vi "Begin.vi"(11 "Image Size":T1=enum."160x120") -> (0 "error out":errorcluster)   [LabVIEW 2012]
doc: "Called before other user functions, this VI is expected to open initial I/O refnums, load in file data, and do all program initialization. Notice that the <B>error out</B> terminal is simply used for data flow. Wiring it to other structures or subVIs ensures that this VI runs first."
uses:
  <vilib>/Rock Robotics/WPI/Camera/WPI_CameraImageSize.ctl
  <vilib>/Rock Robotics/SystemInterfaces/DIO/FPGA_DIOPWMChannel.ctl
  <vilib>/Rock Robotics/WPI/Camera/WPI_CameraWhite Balance Values.ctl
  <vilib>/Rock Robotics/WPI/Camera/WPI_CameraExposure Values.ctl
  <vilib>/Rock Robotics/WPI/Camera/WPI_CameraFrameRate.ctl
  <vilib>/Rock Robotics/WPI/SafetyOutput/WPI_SafetyOutputConfigMenu.ctl
  <vilib>/Rock Robotics/WPI/DriverStation/WPI_DriverStationRobotMode2.ctl
  <vilib>/Rock Robotics/WPI/Joystick/WPI_JoystickDeviceEnum.ctl
  <vilib>/Rock Robotics/SystemInterfaces/Typedef/FPGA_TypedefSolenoidModule.ctl
  <vilib>/Rock Robotics/WPI/Solenoid/WPI_SolenoidChannel.ctl
  <vilib>/Rock Robotics/SystemInterfaces/DIO/FPGA_DIOChannel.ctl
  <vilib>/Rock Robotics/WPI/Encoder/WPI_EncoderType.ctl
  <vilib>/Rock Robotics/SystemInterfaces/Typedef/FPGA_TypedefDigitalModule.ctl
  <vilib>/Rock Robotics/SystemInterfaces/DIO/FPGA_DIORelayChannel.ctl
  <vilib>/Rock Robotics/WPI/RobotDrive/WPI_RobotDriveOpen2MotorWithJaguar.vi
  Robot Global Data.vi
  <vilib>/Rock Robotics/WPI/Solenoid/WPI_SolenoidOpenSingle.vi
  <vilib>/Rock Robotics/WPI/Counter/WPI_CounterDigitalInputToDigitalSource.vi
  <vilib>/Rock Robotics/WPI/MotorControl/WPI_MotorControlOpen Talon.vi
  <vilib>/Rock Robotics/WPI/Compressor/WPI_CompressorGetSetRefNum.vi
panel:
  out "1699-preferences.ini":string[][](array[string])
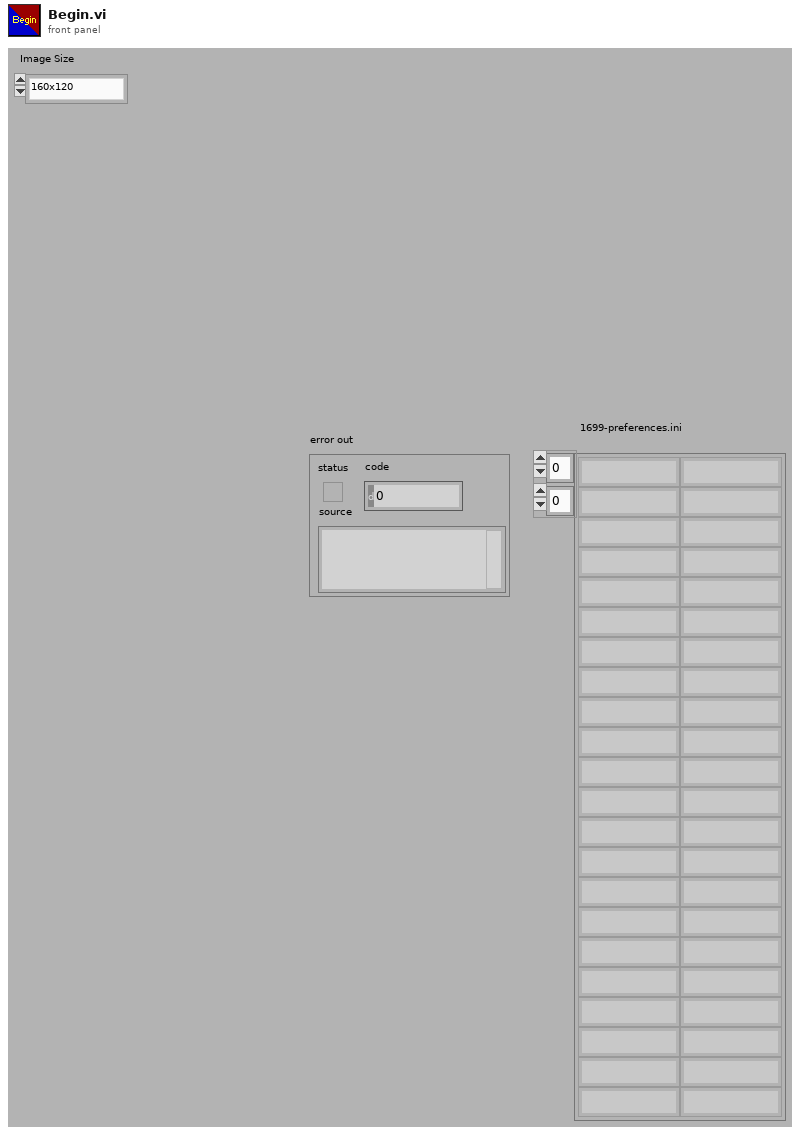
[diagram p1: front panel]
types:
  T1 = typedef "WPI_CameraImageSize.ctl" = enum16{"640x480", "320x240", "160x120"}
  T2 = typedef "FPGA_TypedefDigitalModule.ctl" = enum16{"Digital Module 1", "Digital Module 2"}
  T3 = typedef "FPGA_DIOPWMChannel.ctl" = enum8{"PWM 1", "PWM 2", "PWM 3", "PWM 4", "PWM 5", "PWM 6", "PWM 7", "PWM 8", "PWM 9", "PWM 10", "Invalid"}
  T4 = typedef "FPGA_DIORelayChannel.ctl" = enum8{"Relay 1", "Relay 2", "Relay 3", "Relay 4", "Relay 5", "Relay 6", "Relay 7", "Relay 8", "Invalid"}
  T5 = typedef "FPGA_DIOChannel.ctl" = enum8{"DIO 1", "DIO 2", "DIO 3", "DIO 4", "DIO 5", "DIO 6", "DIO 7", "DIO 8", "DIO 9", "DIO 10", "DIO 11", "DIO 12", "DIO 13", "DIO 14", "Invalid"}
  T6 = typedef "WPI_EncoderType.ctl" = enum16{"1x", "2x", "4x"}
  T7 = typedef "WPI_SolenoidChannel.ctl" = enum8{"Solenoid 1", "Solenoid 2", "Solenoid 3", "Solenoid 4", "Solenoid 5", "Solenoid 6", "Solenoid 7", "Solenoid 8", "Invalid"}
  T8 = typedef "FPGA_TypedefSolenoidModule.ctl" = enum16{"Solenoid Module 1", "Solenoid Module 2"}
  T9 = typedef "WPI_JoystickDeviceEnum.ctl" = enum16{"USB 1", "USB 2", "USB 3", "USB 4", "Kinect 1", "Kinect 2"}
  T10 = typedef "WPI_DriverStationRobotMode2.ctl" = enum16{"Autonomous Disabled", "Autonomous Enabled", "Teleop Disabled", "Teleop Enabled", "Timeout", "Finish", "Test Disabled", "Test Enabled"}
  T11 = typedef "WPI_SafetyOutputConfigMenu.ctl" = enum16{"Enable", "Disable"}
  T12 = typedef "WPI_CameraFrameRate.ctl" = u32
  T13 = typedef "WPI_CameraExposure Values.ctl" = enum16{"Auto", "Flicker-free 50 Hz", "Flicker-free 60 Hz", "Hold current"}
  T14 = typedef "WPI_CameraWhite Balance Values.ctl" = enum16{"Auto", "Fixed indoor", "Fixed outdoor 1", "Fixed outdoor 2", "Fixed fluorescent 1", "Fixed fluorescent 2", "Hold current"}
  T15 = cluster{"[0]":dbl, "[1]":dbl, "[2]":dbl, "[3]":dbl, "[4]":dbl, "[5]":dbl, "[6]":dbl, "[7]":dbl, "[8]":dbl, "[9]":dbl, "[10]":dbl, "[11]":dbl, "[12]":dbl, "[13]":dbl, "[14]":dbl, "[15]":dbl, "[16]":dbl, "[17]":dbl, "[18]":dbl, "[19]":dbl}
  T16 = typedef "WPI_DigitalInputDevRef.ctl" = cluster{"DevStatus":errorcluster, "DIO Channel":T5, "Digital Module":T2}
  T17 = typedef "FPGA_CounterEncoderSourceConvertionLVSourceType.ctl" = cluster{"DevStatus":errorcluster, "AnalogTriggerMode?":bool, "DigitalMode":cluster{"Digital Module":T2, "DIO Channel":T18}, "AnalogTriggerMode":cluster{"AnalogTriggerIndex":T19, "OutputType":T20}}
  T18 = typedef "FPGA_DIODigitalSourceChannel.ctl" = enum8{"DIO 1", "DIO 2", "DIO 3", "DIO 4", "DIO 5", "DIO 6", "DIO 7", "DIO 8", "DIO 9", "DIO 10", "DIO 11", "DIO 12", "DIO 13", "DIO 14", "Disabled"}
  T19 = typedef "FPGA_AnalogTriggerIndex.ctl" = enum8{"Trig 0", "Trig 1", "Trig 2", "Trig 3", "Trig 4", "Trig 5", "Trig 6", "Trig 7", "Invalid"}
  T20 = typedef "FPGA_AnalogTriggerOutType.ctl" = enum16{"InWindow", "TriggerState", "Rising", "Falling"}
  T21 = typedef "WPI_CompressorDevRef.ctl" = cluster{"DevStatus":errorcluster, "DigitalInputDevRef":T16, "RelayDevRef":T22}
  T22 = typedef "WPI_RelayDevRef.ctl" = cluster{"DevStatus":errorcluster, "Relay Channel":T4, "Digital Module":T2, "Relay Direction":T23}
  T23 = typedef "WPI_RelayDirection.ctl" = enum16{"Both directions", "Forward only", "Reverse only"}
  T24 = typedef "WPI_JoystickDevRef.ctl" = cluster{"Device":T9}
  T25 = typedef "WPI_CameraDevRef.ctl" = cluster{"Camera Address":string, "CameraStatus":errorcluster, "Acquire Image Notifier":refnum<notifier>}
  T26 = typedef "WPI_RobotDriveDevRef.ctl" = cluster{"DevStatus":errorcluster, "Motors[]":T27[], "Square Inputs":bool, "Max Output":dbl, "Isochronous":bool}
  T27 = typedef "WPI_MotorControlDeviceRef.ctl" = cluster{"DeviceStatus":errorcluster, "Type":enum16{"PWM", "CAN"}, "PWM":cluster{"Digital Module":T2, "PWM Channel":T3, "DeadBand":T28}, "CAN":cluster{"Device Number":u8, "Control Mode":T29, "Semaphore":T30, "Max Vout":dbl}, "Invert":bool, "TransformRef":T31, "InvTransformRef":T31}
  T28 = typedef "WPI_PWMDeadband.ctl" = cluster{"Name":string, "maxPositivePwm":i32, "minPositivePwm":i32, "centerPwm":i32, "maxNegativePwm":i32, "minNegativePwm":i32, "angularRange":u16}
  T29 = typedef "WPI_CANJaguar_ControlMode.ctl" = enum8{"Percent VBus", "Current", "Speed", "Position", "Voltage"}
  T30 = typedef "Semaphore RefNum" = refnum<k1>
  T31 = typedef "WPI_PWMTransform_ConPane.ctl" = refnum<vi>
  T32 = typedef "WPI_EncoderDevRef.ctl" = cluster{"DevStatus":errorcluster, "EncoderIndex":T33, "CounterIndex":T34, "DistancePerCount":dbl, "Decoding Type":T6}
  T33 = typedef "FPGA_EncoderIdx.ctl" = enum8{"Enc 0", "Enc 1", "Enc 2", "Enc 3", "Invalid"}
  T34 = typedef "FPGA_CounterCtrSystemIndex.ctl" = enum8{"Ctr 0", "Ctr 1", "Ctr 2", "Ctr 3", "Ctr 4", "Ctr 5", "Ctr 6", "Ctr 7", "Invalid"}
  T35 = typedef "WPI_SolenoidDevRef.ctl" = cluster{"DevStatus":errorcluster, "Solenoid Module":T8, "Forward Solenoid Channel":T7, "Reverse Solenoid Channel":T7}
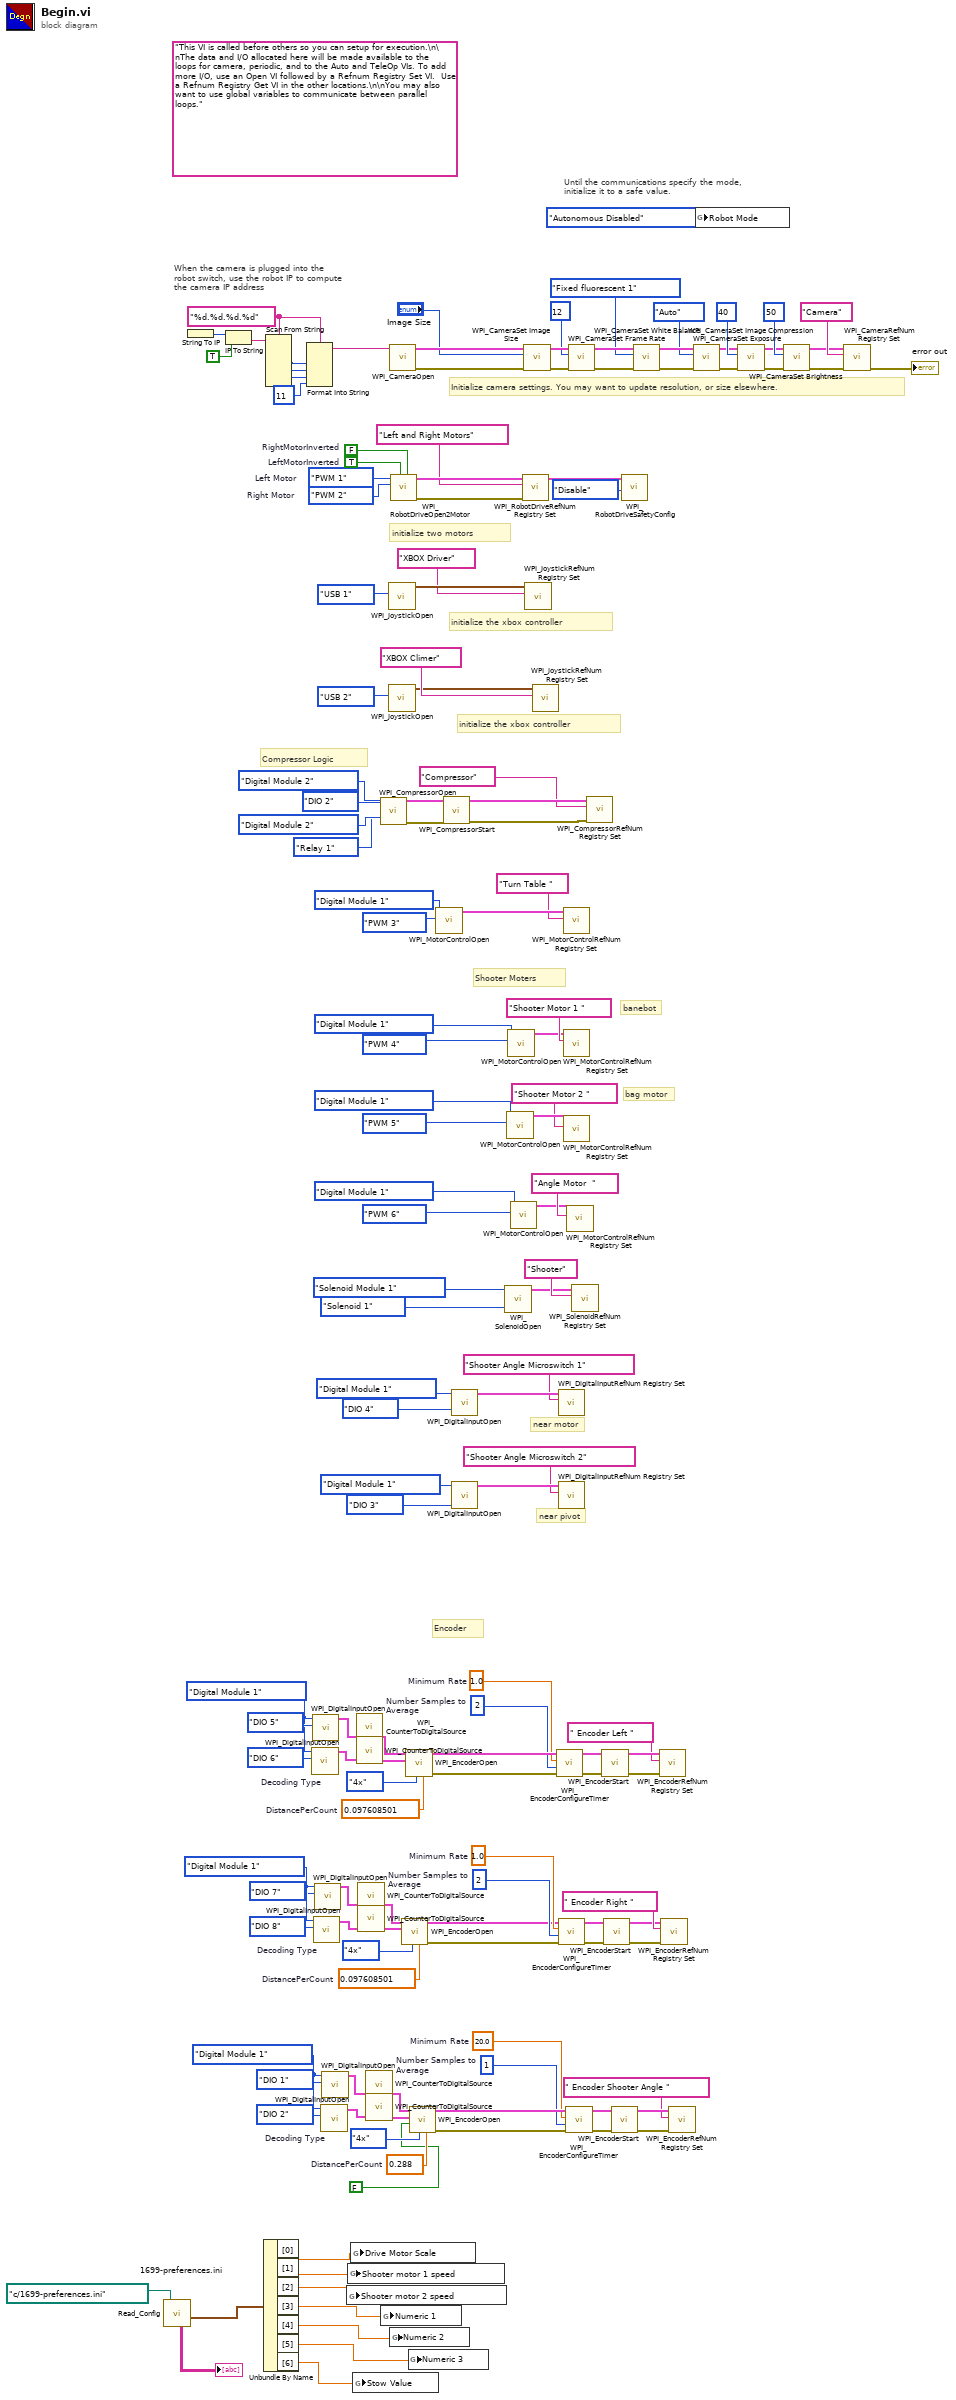
[diagram p0: block diagram]
diagram:
  w45 = FPGA_TypedefDigitalModule."Digital Module 1" ("Digital Module (Module 1)")
  w52 = 0.288  # DistancePerCount
  w53 = WPI_EncoderType."4x"  # Decoding Type
  w54 = u8 1  # Number Samples to Average
  w55 = 20.0  # Minimum Rate
  w80 = FPGA_TypedefDigitalModule."Digital Module 1" ("Digital Module (Module 1)")
  w73 = 0.097608501  # DistancePerCount
  w72 = WPI_EncoderType."4x"  # Decoding Type
  w71 = u8 2  # Number Samples to Average
  w70 = 1.0  # Minimum Rate
  w81 = FPGA_TypedefDigitalModule."Digital Module 1" ("Digital Module (Module 1)")
  w88 = 0.097608501  # DistancePerCount
  w89 = WPI_EncoderType."4x"  # Decoding Type
  w90 = u8 2  # Number Samples to Average
  w91 = 1.0  # Minimum Rate
  w114 = "%d.%d.%d.%d" ("format string")
  (unwired) "This VI is called before others so you can setup for execution.\n\nThe data and I/O allocated here will be made available to the loops for camera, periodic, and to the Auto and TeleOp VIs. To add more I/O, use an Open VI followed by a Refnum Registry Set VI.  Use a Refnum Registry Get VI in the other locations.\n\nYou may also want to use global variables to communicate between parallel loops."
  w125 = FPGA_DIOPWMChannel."PWM 2"  # Right Motor
  w126 = FPGA_DIOPWMChannel."PWM 1"  # Left Motor
  w148 = TRUE  # LeftMotorInverted
  w149 = FALSE  # RightMotorInverted
  # "banebot"
  # "bag motor"
  # "Shooter Moters"
  # "Compressor Logic"
  # "initialize the xbox controller"
  # "near motor"
  # "near pivot"
  # "Encoder"
  # "initialize the xbox controller"
  # "Until the communications specify the mode,\ninitialize it to a safe value."
  # "When the camera is plugged into the\nrobot switch, use the robot IP to compute\nthe camera IP address"
  # "initialize two motors"
  # "Initialize camera settings. You may want to update resolution, or size elsewhere."
  n1 = call "Read_Config.vi"("configuration file path"=path "c:/1699-preferences.ini") -> ("PID Out"=w42:T15, "Array"=→"1699-preferences.ini":string[][])  [unwired: 2 in, 2 out]
  n2 = String To IP() -> (0:w121:u32)  [unwired: 1 in]
  n3 = IP To String(1:TRUE ("dot notation? (F)"), 2:w121) -> (0:w119:string)
  n4 = Unbundle By Name(w42) -> ("[0]"=w41:dbl, "[1]"=w40:dbl, "[2]"=w39:dbl, "[3]"=w38:dbl, "[4]"=w37:dbl, "[5]"=w36:dbl, "[6]"=w35:dbl)
  n5 = Scan From String(format string=w114, input string=w119) -> (output 1=w118:i32, output 2=w117:i32, output 3=w116:i32)  [unwired: 7 in, 3 out]
  n6 = Format Into String(format string=w114, w118, w117, w116, 11 ("Compression")) -> (resulting string=w110:string)  [unwired: 2 in, 1 out]
  n7 = call <vilib>:"WPI_DigitalInputOpen.vi"("DIO Channel"=FPGA_DIOChannel."DIO 6", "Digital Module (Module 1)"=w81) -> ("DigitalInputDevRef"=w85:T16)  [unwired: 8 in, 1 out]
  n8 = call <vilib>:"WPI_DigitalInputOpen.vi"("DIO Channel"=FPGA_DIOChannel."DIO 5", "Digital Module (Module 1)"=w81) -> ("DigitalInputDevRef"=w84:T16)  [unwired: 8 in, 1 out]
  n9 = call <vilib>:"WPI_DigitalInputOpen.vi"("DIO Channel"=FPGA_DIOChannel."DIO 8", "Digital Module (Module 1)"=w80) -> ("DigitalInputDevRef"=w76:T16)  [unwired: 8 in, 1 out]
  n10 = call <vilib>:"WPI_DigitalInputOpen.vi"("DIO Channel"=FPGA_DIOChannel."DIO 7", "Digital Module (Module 1)"=w80) -> ("DigitalInputDevRef"=w77:T16)  [unwired: 8 in, 1 out]
  n11 = call <vilib>:"WPI_DigitalInputOpen.vi"("DIO Channel"=FPGA_DIOChannel."DIO 2", "Digital Module (Module 1)"=w45) -> ("DigitalInputDevRef"=w49:T16)  [unwired: 8 in, 1 out]
  n12 = call <vilib>:"WPI_DigitalInputOpen.vi"("DIO Channel"=FPGA_DIOChannel."DIO 1", "Digital Module (Module 1)"=w45) -> ("DigitalInputDevRef"=w48:T16)  [unwired: 8 in, 1 out]
  n13 = global write "Robot Global Data.vi" "Shooter motor 2 speed"(w39) -> ()
  n14 = global write "Robot Global Data.vi" "Shooter motor 1 speed"(w40) -> ()
  n15 = global write "Robot Global Data.vi" "Drive Motor Scale"(w41) -> ()
  n16 = global write "Robot Global Data.vi" "Stow Value"(w35) -> ()
  n17 = call-poly <vilib>:"WPI_CounterToDigitalSource.vi"("DigitalInputDevRef"=w84) -> ("Digital Source"=w86:T17)  [unwired: 6 in]
  n18 = call-poly <vilib>:"WPI_CounterToDigitalSource.vi"("DigitalInputDevRef"=w85) -> ("Digital Source"=w87:T17)  [unwired: 6 in]
  n19 = call-poly <vilib>:"WPI_CounterToDigitalSource.vi"("DigitalInputDevRef"=w77) -> ("Digital Source"=w75:T17)  [unwired: 6 in]
  n20 = call-poly <vilib>:"WPI_CounterToDigitalSource.vi"("DigitalInputDevRef"=w76) -> ("Digital Source"=w74:T17)  [unwired: 6 in]
  n21 = call-poly <vilib>:"WPI_CounterToDigitalSource.vi"("DigitalInputDevRef"=w48) -> ("Digital Source"=w50:T17)  [unwired: 6 in]
  n22 = call-poly <vilib>:"WPI_CounterToDigitalSource.vi"("DigitalInputDevRef"=w49) -> ("Digital Source"=w51:T17)  [unwired: 6 in]
  n23 = call <vilib>:"WPI_CompressorOpen.vi"("Pressure Switch Digital Module (Module 1)"=FPGA_TypedefDigitalModule."Digital Module 2", "Pressure Switch DIO Channel"=FPGA_DIOChannel."DIO 2", "Relay Digital Module (Module 1)"=FPGA_TypedefDigitalModule."Digital Module 2", "Relay Channel"=FPGA_DIORelayChannel."Relay 1") -> ("CompressorDevRef"=w26:T21, "error out"=w25:errorcluster)  [unwired: 10 in]
  n24 = global write "Robot Global Data.vi" "Numeric 1"(w38) -> ()
  n25 = call <vilib>:"WPI_JoystickOpen.vi"("JoystickDevice"=WPI_JoystickDeviceEnum."USB 1") -> ("JoystickDevRef"=w105:T24)  [unwired: 10 out]
  n26 = call <vilib>:"WPI_JoystickOpen.vi"("JoystickDevice"=WPI_JoystickDeviceEnum."USB 2") -> ("JoystickDevRef"=w106:T24)  [unwired: 10 out]
  n27 = call <vilib>:"WPI_CameraOpen.vi"("Camera Address"=w110) -> ("error out"=w135:errorcluster, "CameraDevRef"=w136:T25)  [unwired: 1 in, 8 out]
  n28 = global write "Robot Global Data.vi" "Numeric 2"(w37) -> ()
  n29 = call-poly <vilib>:"WPI_RobotDriveOpen2Motor.vi"("Right Motor Inverted"=w149, "Left Motor Inverted"=w148, "Right Motor"=w125, "Left Motor"=w126) -> ("error out"=w144:errorcluster, "RobotDriveDevRef"=w146:T26)  [unwired: 1 in, 5 out]
  n30 = call <vilib>:"WPI_EncoderOpen.vi"("DistancePerCount"=w73, "Decoding Type"=w72, "BSource"=w74, "ASource"=w75) -> ("error out"=w69:errorcluster, "EncoderDevRef"=w63:T32)  [unwired: 6 in]
  n31 = call <vilib>:"WPI_EncoderOpen.vi"("DistancePerCount"=w88, "Decoding Type"=w89, "BSource"=w87, "ASource"=w86) -> ("error out"=w92:errorcluster, "EncoderDevRef"=w98:T32)  [unwired: 6 in]
  n32 = global write "Robot Global Data.vi" "Numeric 3"(w36) -> ()
  n33 = call <vilib>:"WPI_EncoderOpen.vi"("DistancePerCount"=w52, "Decoding Type"=w53, "Invert Direction (False)"=FALSE, "BSource"=w51, "ASource"=w50) -> ("error out"=w56:errorcluster, "EncoderDevRef"=w62:T32)  [unwired: 5 in]
  n34 = call-poly <vilib>:"WPI_MotorControlOpen.vi"("PWM Channel"=FPGA_DIOPWMChannel."PWM 3", "Digital Module (Module 1)"=FPGA_TypedefDigitalModule."Digital Module 1") -> ("MotorControlDeviceRef"=w16:T27)  [unwired: 8 in, 1 out]
  n35 = call <vilib>:"WPI_CompressorStart.vi"("error in (no error)"=w25, "CompressorDevRef"=w26) -> ("error out"=w24:errorcluster, "CompressorDevRef"=w23:T21)  [unwired: 8 in]
  n36 = call <vilib>:"WPI_DigitalInputOpen.vi"("DIO Channel"=FPGA_DIOChannel."DIO 4", "Digital Module (Module 1)"=FPGA_TypedefDigitalModule."Digital Module 1") -> ("DigitalInputDevRef"=w29:T16)  [unwired: 1 in, 8 out]
  n37 = call <vilib>:"WPI_DigitalInputOpen.vi"("DIO Channel"=FPGA_DIOChannel."DIO 3", "Digital Module (Module 1)"=FPGA_TypedefDigitalModule."Digital Module 1") -> ("DigitalInputDevRef"=w30:T16)  [unwired: 1 in, 8 out]
  n38 = call-poly <vilib>:"WPI_SolenoidOpen.vi"("Solenoid Channel"=WPI_SolenoidChannel."Solenoid 1", "Solenoid Module (Module 1)"=FPGA_TypedefSolenoidModule."Solenoid Module 1") -> ("SolenoidDevRef"=w99:T35)  [unwired: 8 in, 1 out]
  n39 = call-poly <vilib>:"WPI_MotorControlOpen.vi"("PWM Channel"=FPGA_DIOPWMChannel."PWM 5", "Digital Module (Module 1)"=FPGA_TypedefDigitalModule."Digital Module 1") -> ("MotorControlDeviceRef"=w11:T27)  [unwired: 8 in, 1 out]
  n40 = call-poly <vilib>:"WPI_MotorControlOpen.vi"("PWM Channel"=FPGA_DIOPWMChannel."PWM 4", "Digital Module (Module 1)"=FPGA_TypedefDigitalModule."Digital Module 1") -> ("MotorControlDeviceRef"=w8:T27)  [unwired: 8 in, 1 out]
  n41 = call-poly <vilib>:"WPI_MotorControlOpen.vi"("PWM Channel"=FPGA_DIOPWMChannel."PWM 6", "Digital Module (Module 1)"=FPGA_TypedefDigitalModule."Digital Module 1") -> ("MotorControlDeviceRef"=w3:T27)  [unwired: 8 in, 1 out]
  n42 = call <vilib>:"WPI_RobotDriveRefNum Registry Set.vi"("error in (no error)"=w144, "refnum name"="Left and Right Motors", "RobotDriveDevRef"=w146) -> ("RobotDriveDevRef"=w113:T26)  [unwired: 8 out]
  n43 = call <vilib>:"WPI_CameraSet Image Size.vi"("error in (no error)"=w135, "Image Size"="Image Size", "CameraDevRef"=w136) -> ("error out"=w134:errorcluster, "CameraDevRef Out"=w137:T25)  [unwired: 7 out]
  n44 = call <vilib>:"WPI_JoystickRefNum Registry Set.vi"("refnum name"="XBOX Driver", "JoystickDevRef"=w105) -> ()  [unwired: 1 in, 9 out]
  n45 = call <vilib>:"WPI_JoystickRefNum Registry Set.vi"("refnum name"="XBOX Climer", "JoystickDevRef"=w106) -> ()  [unwired: 1 in, 9 out]
  n46 = call <vilib>:"WPI_EncoderConfigureTimer.vi"("error in (no error)"=w92, "Number Samples to Average"=w90, "Minimum Rate"=w91, "EncoderDevRef"=w98) -> ("error out"=w93:errorcluster, "EncoderDevRef"=w97:T32)  [unwired: 6 in]
  n47 = call <vilib>:"WPI_DigitalInputRefNum Registry Set.vi"("refnum name"="Shooter Angle Microswitch 1", "DigitalInputDevRef"=w29) -> ()  [unwired: 8 in, 2 out]
  n48 = call <vilib>:"WPI_DigitalInputRefNum Registry Set.vi"("refnum name"="Shooter Angle Microswitch 2", "DigitalInputDevRef"=w30) -> ()  [unwired: 8 in, 2 out]
  n49 = call <vilib>:"WPI_EncoderConfigureTimer.vi"("error in (no error)"=w69, "Number Samples to Average"=w71, "Minimum Rate"=w70, "EncoderDevRef"=w63) -> ("error out"=w68:errorcluster, "EncoderDevRef"=w64:T32)  [unwired: 6 in]
  n50 = call <vilib>:"WPI_MotorControlRefNum Registry Set.vi"("refnum name"="Turn Table ", "MotorControlDevRef"=w16) -> ()  [unwired: 8 in, 2 out]
  n51 = call <vilib>:"WPI_MotorControlRefNum Registry Set.vi"("refnum name"="Shooter Motor 1 ", "MotorControlDevRef"=w8) -> ()  [unwired: 8 in, 2 out]
  n52 = call <vilib>:"WPI_MotorControlRefNum Registry Set.vi"("refnum name"="Shooter Motor 2 ", "MotorControlDevRef"=w11) -> ()  [unwired: 8 in, 2 out]
  n53 = call <vilib>:"WPI_EncoderConfigureTimer.vi"("error in (no error)"=w56, "Number Samples to Average"=w54, "Minimum Rate"=w55, "EncoderDevRef"=w62) -> ("error out"=w57:errorcluster, "EncoderDevRef"=w61:T32)  [unwired: 6 in]
  n54 = call <vilib>:"WPI_MotorControlRefNum Registry Set.vi"("refnum name"="Angle Motor  ", "MotorControlDevRef"=w3) -> ()  [unwired: 8 in, 2 out]
  n55 = call <vilib>:"WPI_CameraSet Frame Rate.vi"("error in (no error)"=w134, "Frame Rate (fps)"=T12 12, "CameraDevRef"=w137) -> ("error out"=w133:errorcluster, "CameraDevRef Out"=w139:T25)  [unwired: 7 out]
  n56 = call <vilib>:"WPI_SolenoidRefNum Registry Set.vi"("refnum name"="Shooter", "SolenoidDevRef"=w99) -> ()  [unwired: 8 in, 2 out]
  n57 = call <vilib>:"WPI_CompressorRefNum Registry Set.vi"("error in (no error)"=w24, "refnum name"="Compressor", "CompressorDevRef"=w23) -> ()  [unwired: 7 in, 2 out]
  n58 = call <vilib>:"WPI_EncoderStart.vi"("error in (no error)"=w93, "EncoderDevRef"=w97) -> ("error out"=w94:errorcluster, "EncoderDevRef"=w96:T32)  [unwired: 8 in]
  n59 = call <vilib>:"WPI_EncoderStart.vi"("error in (no error)"=w68, "EncoderDevRef"=w64) -> ("error out"=w67:errorcluster, "EncoderDevRef"=w65:T32)  [unwired: 8 in]
  n60 = call <vilib>:"WPI_EncoderStart.vi"("error in (no error)"=w57, "EncoderDevRef"=w61) -> ("error out"=w58:errorcluster, "EncoderDevRef"=w60:T32)  [unwired: 8 in]
  n61 = call <vilib>:"WPI_RobotDriveSafetyConfig.vi"("mode"=WPI_SafetyOutputConfigMenu."Disable", "RobotDriveDevRef"=w113) -> ()  [unwired: 8 in, 2 out]
  n62 = call <vilib>:"WPI_CameraSet White Balance.vi"("error in (no error)"=w133, "White Balance"=WPI_CameraWhite_Balance_Values."Fixed fluorescent 1", "CameraDevRef"=w139) -> ("error out"=w132:errorcluster, "CameraDevRef Out"=w138:T25)  [unwired: 7 out]
  n63 = call <vilib>:"WPI_EncoderRefNum Registry Set.vi"("error in (no error)"=w94, "refnum name"=" Encoder Left ", "EncoderDevRef"=w96) -> ()  [unwired: 7 in, 2 out]
  n64 = call <vilib>:"WPI_EncoderRefNum Registry Set.vi"("error in (no error)"=w67, "refnum name"=" Encoder Right ", "EncoderDevRef"=w65) -> ()  [unwired: 7 in, 2 out]
  n65 = call <vilib>:"WPI_EncoderRefNum Registry Set.vi"("error in (no error)"=w58, "refnum name"=" Encoder Shooter Angle ", "EncoderDevRef"=w60) -> ()  [unwired: 7 in, 2 out]
  n66 = call <vilib>:"WPI_CameraSet Exposure.vi"("error in (no error)"=w132, "Exposure"=WPI_CameraExposure_Values."Auto", "CameraDevRef"=w138) -> ("error out"=w131:errorcluster, "CameraDevRef Out"=w141:T25)  [unwired: 7 out]
  n67 = global write "Robot Global Data.vi" "Robot Mode"(WPI_DriverStationRobotMode2."Autonomous Disabled" ("Robot Mode")) -> ()
  n68 = call <vilib>:"WPI_CameraSet Image Compression.vi"("error in (no error)"=w131, "Compression"=40, "CameraDevRef"=w141) -> ("error out"=w130:errorcluster, "CameraDevRef Out"=w140:T25)  [unwired: 7 out]
  n69 = call <vilib>:"WPI_CameraSet Brightness.vi"("error in (no error)"=w130, "Brightness"=50, "CameraDevRef"=w140) -> ("error out"=w128:errorcluster, "CameraDevRef Out"=w129:T25)  [unwired: 7 out]
  n70 = call <vilib>:"WPI_CameraRefNum Registry Set.vi"("error in (no error)"=w128, "refnum name"="Camera", "CameraDevRef"=w129) -> ("error out"=→"error out":errorcluster)  [unwired: 8 out]
